vi "Initialise.vi"(8 "error in (no error)":errorcluster, 10 "Message in":refnum<class "InitialiseMessage.lvclass">, 11 "ServiceManager in":refnum<class "ServiceManager.lvclass">) -> (0 "error out":errorcluster, 3 "ServiceManager out":refnum<class "ServiceManager.lvclass">)   [LabVIEW 2012, in "ServiceManager.lvclass"]
uses:
  ServiceManager.lvclass
  <vilib>/Distrio/Murmex/InitialiseMessage/InitialiseMessage.lvclass
  <vilib>/Utility/miscctls.llb/LVPointTypeDef.ctl
  <vilib>/Distrio/Murmex/Murmex/Murmex.lvclass
  ServiceManager.lvclass/ServiceManager.ctl
  loaded_components_cluster.ctl
  <vilib>/Distrio/Murmex/Murmex/component_specification_cluster.ctl
  <vilib>/Distrio/Murmex/Murmex/status_enum.ctl
  <vilib>/Distrio/Murmex/TerminateMessage/TerminateMessage.lvclass
  <vilib>/Distrio/Murmex/InspectMessage/InspectMessage.lvclass
  <vilib>/Distrio/Murmex/Murmex/Get VI reference.vi
  <vilib>/Distrio/Murmex/Murmex/Set VI reference.vi
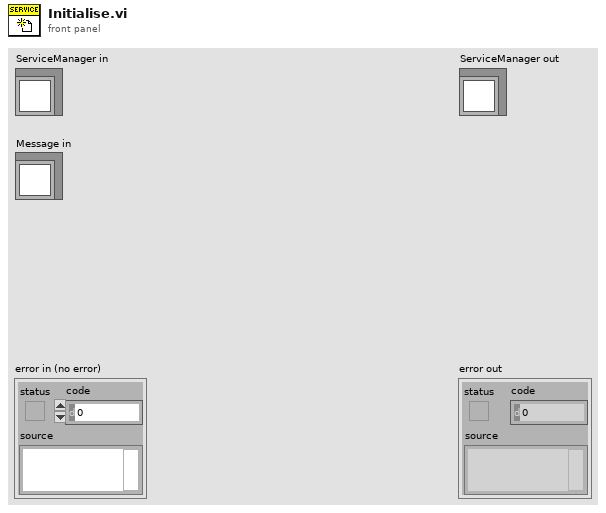
[diagram p1: front panel]
types:
  T1 = typedef "LVPointTypeDef.ctl" = cluster{"Horizontal":i16, "Vertical":i16}
  T2 = cluster{"button:config locally ref":refnum<vi>, "button:check existence":refnum<vi>, "button:kill_comp":refnum<vi>, "button:restart_comp":refnum<vi>}
  T3 = typedef "Murmex.lvlib/Murmex.lvclass/status_enum.ctl" = enum16{"ready", "warning", "error", "shutting down", "initialising"}
  T4 = typedef "ServiceManager.lvclass/loaded_components_cluster.ctl" = cluster{"component specification":T5, "booted?":bool, "status":T3, "last seen?":timestamp}
  T5 = typedef "Murmex.lvlib/Murmex.lvclass/component_specification_cluster.ctl" = cluster{"name":string, "language":string, "host name":string, "id":string}
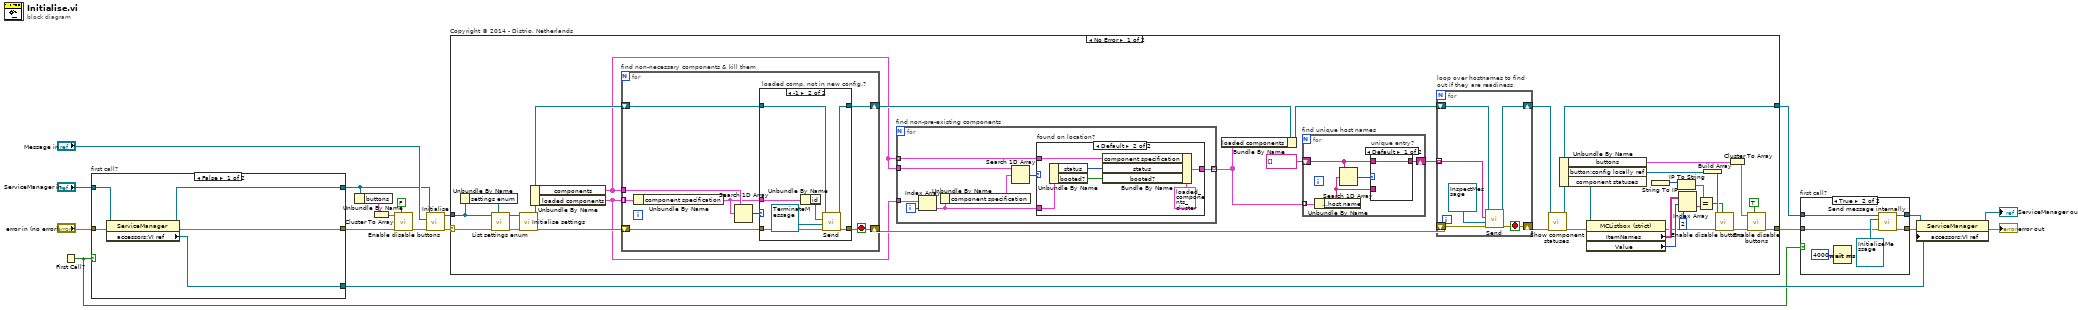
[diagram p0: block diagram]
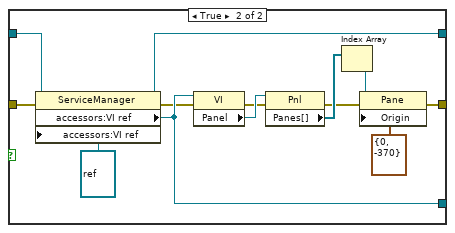
[diagram p3: hidden frame]
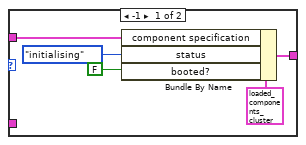
[diagram p4: hidden frame]
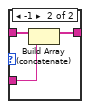
[diagram p6: hidden frame]
diagram:
  n1 = First Call?() -> (First Call?: T/F=w3:bool)
  n2 = case "first call?" shown="False" w3 {
    tunnel: "ServiceManager in" -> [w24 w37]
    tunnel: "error in (no error)" -> [w23 w36]
    tunnel: [w22 w25] -> w11
    tunnel: [w21 w35] -> w9
    tunnel: [w20 w33] -> w8
    frame False {
      n3 = property class="ServiceManager"(reference=w24, error in=w23) -> (reference out=w21:refnum<class "ServiceManager.lvclass">, error out=w22:errorcluster, "accessors:VI ref"=w20:refnum<vi>)
    }
    frame True {
      n4 = property class="ServiceManager"(reference=w37, error in=w36, "accessors:VI ref"=refnum<vi> refnum ("VI ref")) -> (reference out=w35:refnum<class "ServiceManager.lvclass">, error out=w32:errorcluster, "accessors:VI ref"=w33:refnum<vi>)
      n5 = property class="VI"(reference=w33, error in=w32) -> (error out=w30:errorcluster, "Panel"=w31:refnum<vi>)  [unwired: 1 out]
      n6 = property class="Pnl"(reference=w31, error in=w30) -> (error out=w26:errorcluster, "Panes[]"=w29:refnum<vi>[])  [unwired: 1 out]
      n7 = Index Array(array=w29) -> (element=w28:refnum<vi>)  [unwired: 1 in]
      n8 = property class="Pane"(reference=w28, error in=w26, "Origin"=T1 {"Horizontal"=0, "Vertical"=-370}) -> (error out=w25:errorcluster)  [unwired: 1 out]
    }
  }
  n9 = Unbundle By Name(w9) -> ("buttons"=w14:T2)
  n10 = Cluster To Array(cluster=w14) -> (array=w16:refnum<vi>[])
  n11 = call "Enable disable buttons.vi"("enable?"=FALSE, "error in (no error)"=w11, "references"=w16) -> ("error out"=w13:errorcluster)  [unwired: 8 in]
  n12 = call-parent "Initialise.vi"("error in (no error)"=w13, "Message in"="Message in", "Murmex in"=w9) -> ("error out"=w19:errorcluster, "Murmex out"=w18:refnum<class "ServiceManager.lvclass">)  [unwired: 7 in]
  n13 = case "Copyright © 2014 - Distrio, Netherlands" shown="No Error" w19 {
    selector: w19 -> [w46 w125]
    tunnel: w18 -> [w47 w124]
    tunnel: [w42 w125] -> w5
    tunnel: [w49 w124] -> w2
    frame No Error {
      n14 = Unbundle By Name(w47) -> ("settings enum"=w64:refnum<vi>)
      n15 = call-dynamic "List settings enum.vi"("setting enum reference"=w64, "error in (no error)"=w46, "ServiceManager in"=w47) -> ("error out"=w65:errorcluster, "ServiceManager out"=w66:refnum<class "ServiceManager.lvclass">)  [unwired: 7 in]
      n16 = call-dynamic "Initialise settings.vi"("error in (no error)"=w65, "ServiceManager in"=w66) -> ("error out"=w67:errorcluster, "ServiceManager out"=w41:refnum<class "ServiceManager.lvclass">)  [unwired: 8 in]
      n17 = Unbundle By Name(w41) -> ("components"=w39:T5[], "loaded components"=w38:T4[])
      n18 = for "find non-necessary components & kill them" {
        tunnel: w39 -> [w99]
        shift-right: [w95] -> w69
        shift-left: w67 -> [w98]
        tunnel: w38 -> [w93] mode=indexing
        shift-right: [w92] -> w40
        shift-left: w41 -> [w94]
        stop <- w95 stop-if-true
        n19 = Unbundle By Name(w93) -> ("component specification"=w97:T5)
        n20 = Search 1D Array(1D array=w99, element=w97) -> (index of element=w96:i32)  [unwired: 1 in]
        n21 = case "loaded comp. not in new config.?" shown="-1" w96 {
          tunnel: w97 -> [_ w108]
          tunnel: [w101 w106] -> w95
          tunnel: w98 -> [w101 w104]
          tunnel: w94 -> [w100 w105]
          tunnel: [w100 w102] -> w92
          frame Default {
          }
          frame -1 {
            n22 = Unbundle By Name(w108) -> ("id"=w107:string)
            n23 = call <vilib>:"Send.vi"("error in (no error)"=w104, "Message"=refnum<class "TerminateMessage.lvclass"> refnum ("TerminateMessage.lvclass"), "recipient"=w107, "Murmex in"=w105) -> ("error out"=w106:errorcluster, "Murmex out"=w102:refnum<class "ServiceManager.lvclass">)  [unwired: 6 in]
          }
        }
      }
      n24 = for "find non-pre-existing components" {
        tunnel: w38 -> [w80]
        tunnel: w39 -> [w78]
        tunnel: w39 -> [w76] mode=indexing
        tunnel: [w75] -> w68 mode=indexing
        i -> [w77]
        n25 = Index Array(array=w80, index=w77) -> (element=w73:T4)
        n26 = Unbundle By Name(w73) -> ("component specification"=w74:T5)
        n27 = Search 1D Array(1D array=w78, element=w74) -> (index of element=w79:i32)  [unwired: 1 in]
        n28 = case "found on location?" shown="Default" w79 {
          tunnel: w76 -> [w85 w91]
          tunnel: [w82 w89] -> w75
          tunnel: w73 -> [_ w88]
          frame -1 {
            n29 = Bundle By Name(cluster=T4 {"component specification"={"name"="", "language"="", "host name"="", "id"=""}, "booted?"=FALSE, "status"=enum."ready", "last seen?"=timestamp(0 s since 1904-01-01)} ("component"), "component specification"=w85, "status"=status_enum."initialising", "booted?"=FALSE ("ready?")) -> (w82:T4)
          }
          frame Default {
            n30 = Unbundle By Name(w88) -> ("status"=w87:T3, "booted?"=w86:bool)
            n31 = Bundle By Name(cluster=T4 {"component specification"={"name"="", "language"="", "host name"="", "id"=""}, "booted?"=FALSE, "status"=enum."ready", "last seen?"=timestamp(0 s since 1904-01-01)} ("component"), "component specification"=w91, "status"=w87, "booted?"=w86) -> (w89:T4)
          }
        }
      }
      n32 = Bundle By Name(cluster=w40, "loaded components"=w68) -> (w70:refnum<class "ServiceManager.lvclass">)
      n33 = for "find unique host names" {
        tunnel: w68 -> [w113] mode=indexing
        shift-right: [w112] -> w71
        shift-left: string[] [] -> [w111]
        n34 = Unbundle By Name(w113) -> ("component specification.host name"=w110:string)
        n35 = Search 1D Array(1D array=w111, element=w110) -> (index of element=w109:i32)  [unwired: 1 in]
        n36 = case "unique entry?" shown="Default" w109 {
          tunnel: [w114 w117] -> w112
          tunnel: w111 -> [w114 w116]
          tunnel: w110 -> [_ w115]
          frame Default {
          }
          frame -1 {
            n37 = Build Array (concatenate)(w116, w115) -> (w117:string[])
          }
        }
      }
      n38 = for "loop over hostnames to find \nout if they are readiness" {
        shift-right: [w123] -> w51
        shift-left: w69 -> [w118]
        tunnel: w71 -> [w120] mode=indexing
        shift-right: [w121] -> w52
        shift-left: w70 -> [w122]
        stop <- w123 stop-if-true
        n39 = call <vilib>:"Send.vi"("error in (no error)"=w118, "Message"=refnum<class "InspectMessage.lvclass"> refnum ("InspectMessage.lvclass"), "recipient"=w120, "Murmex in"=w122) -> ("error out"=w123:errorcluster, "Murmex out"=w121:refnum<class "ServiceManager.lvclass">)  [unwired: 6 in]
      }
      n40 = call-dynamic "Show component statuses.vi"("error in (no error)"=w51, "ServiceManager in"=w52) -> ("error out"=w50:errorcluster, "ServiceManager out"=w49:refnum<class "ServiceManager.lvclass">)  [unwired: 8 in]
      n41 = Unbundle By Name(w49) -> ("buttons"=w43:T2, "button:config locally ref"=w55:refnum<vi>, "component statuses"=w63:refnum<vi>)
      n42 = property class="MCListbox (strict)"(reference=w63, error in=w50) -> (error out=w54:errorcluster, "ItemNames"=w58:string[][], "Value"=w59:i32)  [unwired: 1 out]
      n43 = String To IP ("local IP")() -> (0:w60:u32)  [unwired: 1 in]
      n44 = IP To String(2:w60) -> (0:w61:string)  [unwired: 1 in]
      n45 = Index Array(array=w58, index (row)=w59, index (col)=2 ("disabled index (col)")) -> (element=w62:string)
      n46 = Equal?(x=w61, y=w62) -> (x = y?=w53:bool)
      n47 = Build Array(w55) -> (w56:refnum<vi>[])
      n48 = call "Enable disable buttons.vi"("enable?"=w53, "error in (no error)"=w54, "references"=w56) -> ("error out"=w48:errorcluster)  [unwired: 8 in]
      n49 = Cluster To Array(cluster=w43) -> (array=w44:refnum<vi>[])
      n50 = call "Enable disable buttons.vi"("enable?"=TRUE, "error in (no error)"=w48, "references"=w44) -> ("error out"=w42:errorcluster)  [unwired: 8 in]
    }
    frame Error {
    }
  }
  n51 = case "first call?" shown="True" w3 {
    tunnel: [w127 w129] -> w4
    tunnel: w5 -> [w127 w130]
    tunnel: w2 -> [w126 w131]
    tunnel: [w126 w128] -> w1
    frame False {
    }
    frame True {
      n52 = Wait (ms)(milliseconds to wait=u32 4000) -> ()  [unwired: 1 out]
      n53 = call <vilib>:"Send message internally.vi"("error in (no error)"=w130, "Message"=refnum<class "InitialiseMessage.lvclass"> refnum ("Distrio Murmex 1.5:InitialiseMessage"), "Murmex in"=w131) -> ("error out"=w129:errorcluster, "Murmex out"=w128:refnum<class "ServiceManager.lvclass">)  [unwired: 7 in]
    }
  }
  n54 = property class="ServiceManager"(reference=w1, error in=w4, "accessors:VI ref"=w8) -> (reference out=→"ServiceManager out":refnum<class "ServiceManager.lvclass">, error out=→"error out":errorcluster)
